vi "PID_linear.vi"(8 "Stop Controller Loop":bool) -> ()   [LabVIEW 2017]
uses:
  <vilib>/Platform/TimedLoop/XDataNode/timing_clust.ctl
  <vilib>/Platform/TimedLoop/XDataNode/nitl_modes.ctl
  <vilib>/Platform/TimedLoop/XDataNode/wakeup.ctl
  <vilib>/platform/TimedLoop/XDataNode/XDataNode.xnode
  <vilib>/Platform/TimedLoop/XDataNode/XDNodeRunTimeDep.lvlib
panel:
  in  "Starting Actuation State":dbl
  out "PID Actuations":dbl[](graph)
  in  "Actuation Min":dbl
  in  "Actuation Max":dbl
  out "Error":dbl
  out "Feedback":dbl
  out "Setpoint":dbl
  out "Saturated":bool
  out "Derivative State":dbl
  in  "Step Smoothing":dbl
  in  "Derivitative Max":dbl
  in  "D Gain":dbl
  out "Anti Windup":bool
  out "Integrator State":dbl
  in  "Integrator Min":dbl
  in  "Integrator Max":dbl
  in  "I Gain":dbl
  in  "P Gain":dbl
  # "PID Control"
  # "Proportional Control"
  # "Actuation Limits"
  # "Anti Windup Strategy"
  # "If the calcuated Actuation exceeds the Actuation Max or the Actuation Min, the Integrator State will only be allowed to accumulate in the direction of the allowed Actuation range and the Actuation will be saturated.\n\nIf the calculated Integrator State will be saturated to either the Integrator Max or Integrator Min."
  # "Integral Control"
  # "Integral Control"
  # "Derivative Smoothing Strategy"
  # "The derivative is calculated every n steps provide in the Step Smoothing Numeric Control for derivative smoothing."
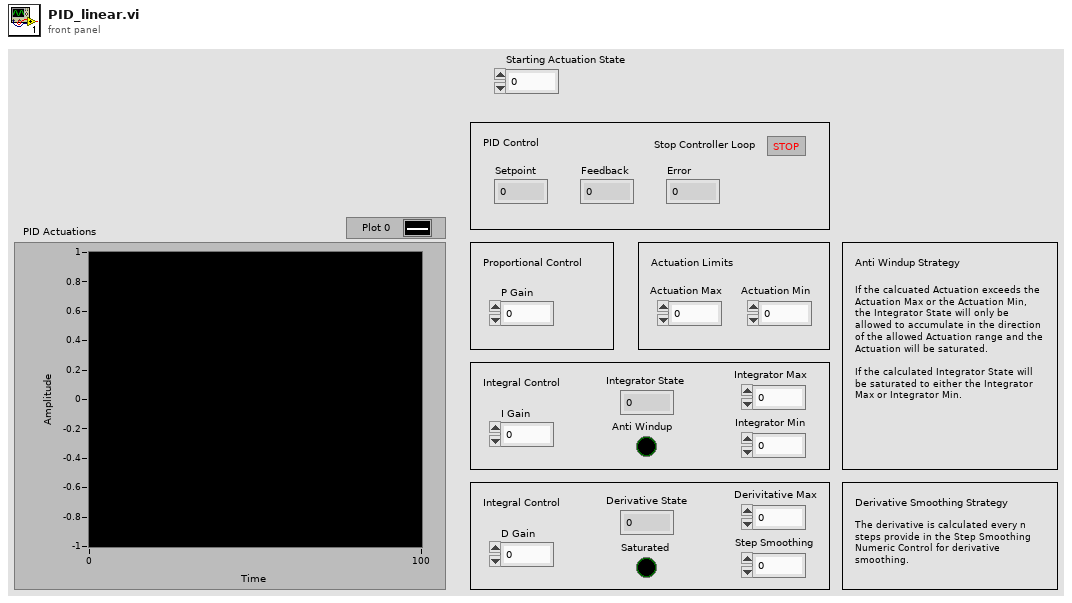
[diagram p1: front panel]
types:
  T1 = typedef "XDNodeRunTimeDep.lvlib/timing_clust.ctl" = cluster{"Expected End [f-1]":u64, "Actual End [f-1]":u64, "Finished Late? [f-1]":bool, "Expected End [i-1]":u64, "Actual End [i-1]":u64, "Finished Late? [i-1]":bool, "Expected Start [i]":u64, "Actual Start [i]":u64, "Expected Start [f]":u64, "Actual Start [f]":u64, "Source Name":string, "Structure Name":string, "Period":i64, "Deadline":i64, "Offset":i64, "Start":i64, "Priority":i32, "Timeout":i32, "Mode":T2, "Wakeup Reason":T3, "Error":errorcluster, "Source Type":string, "Secondary Source Type":string, "Global End Time":u64, "Global Start Time":u64, "Frame Duration":u64, "Iteration Duration":u64, "Assigned CPU":i32, "I/O Scan Engine Mode":u32}
  T2 = typedef "XDNodeRunTimeDep.lvlib/nitl_modes.ctl" = enum32{"No Change", "Process missed periods, maintain original phase", "Discard missed periods, maintain original phase", "Process missed periods, ignore original phase", "Discard missed periods, ignore original phase"}
  T3 = typedef "XDNodeRunTimeDep.lvlib/wakeup.ctl" = enum32{"Normal", "Aborted", "Asynchronous wakeup", "Timing source error", "Timed loop error", "Timeout"}
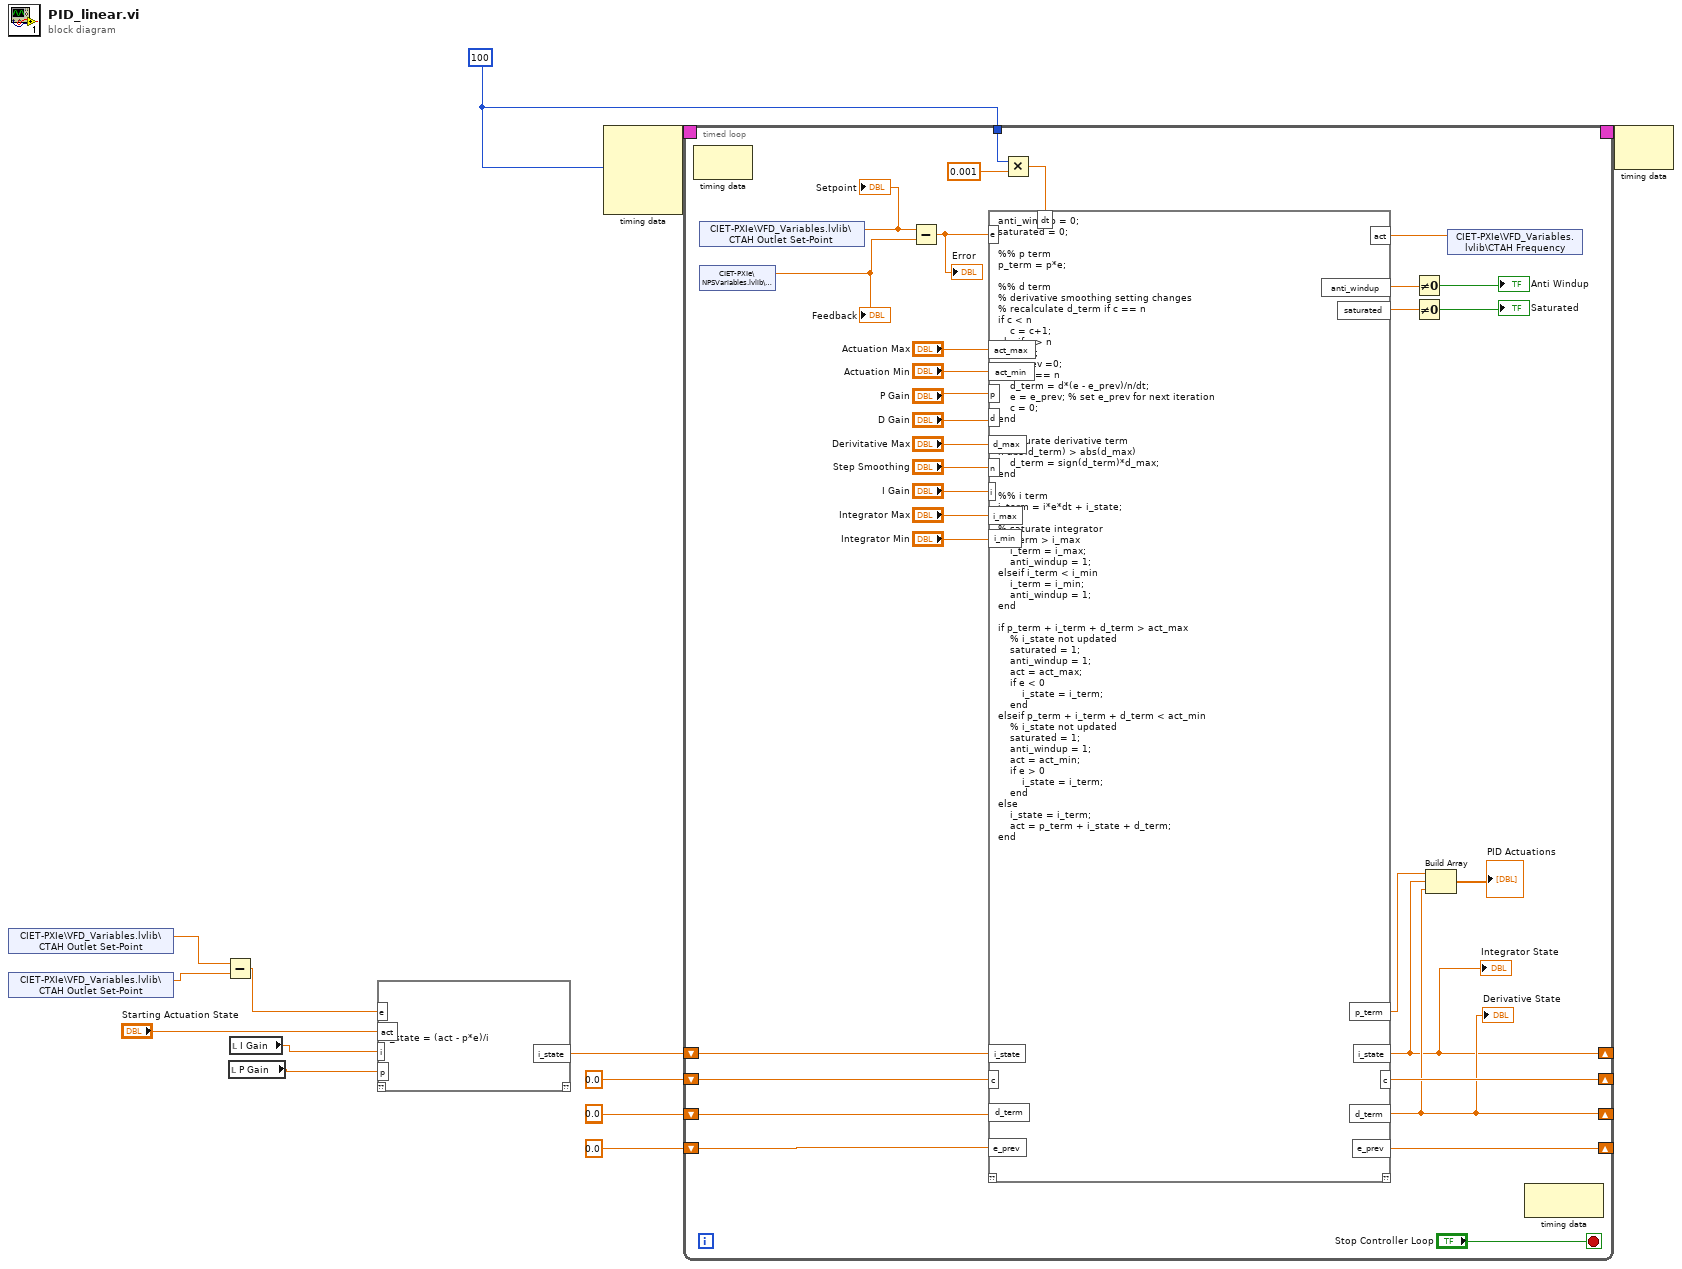
[diagram p0: block diagram]
diagram:
  w8 = 100
  (unwired) 0.0
  n1 = shared-variable "CIET-PXIe\\VFD_Variables.lvlib\\CTAH Outlet Set-Point"() -> (w4:dbl)  [unwired: 1 in, 1 out]
  n2 = shared-variable "CIET-PXIe\\VFD_Variables.lvlib\\CTAH Outlet Set-Point"() -> (w5:dbl)  [unwired: 1 in, 1 out]
  n3 = Subtract(x=w4, y=w5) -> (x-y=w3:dbl)
  n4 = local read "P Gain"() -> (w2:dbl)
  n5 = local read "I Gain"() -> (w1:dbl)
  n6 = script code="i_state = (act - p*e)/i"("e"=w3, "i"=w1, "act"="Starting Actuation State", "p"=w2) -> ("i_state"=w6:dbl)  [unwired: 1 in, 1 out]
  n7 = node-c288(w8) -> (w13:T1)  [unwired: 3 in]
  n8 = timed-loop {
    timing: w13 -> [_]
    timing-out: [_] -> w12
    shift-right: [w24] -> _
    shift-left: w6 -> [w33]
    shift-right: [w28] -> _
    shift-left: 0.0 -> [w32]
    shift-right: [w25] -> _
    shift-left: 0.0 -> [w31]
    shift-right: [w29] -> _
    shift-left: 0.0 -> [w30]
    tunnel: w8 -> [w20]
    stop <- "Stop Controller Loop" stop-if-true
    n9 = node-c288() -> ()  [unwired: 1 in, 1 out]
    n10 = shared-variable "CIET-PXIe\\VFD_Variables.lvlib\\CTAH Outlet Set-Point"() -> (w15:dbl)  [unwired: 1 in, 1 out]
    "Setpoint" <- w15
    n11 = shared-variable "CIET-PXIe\\NPSVariables.lvlib\\BT-41"() -> (w14:sgl)  [unwired: 1 in, 1 out]
    "Feedback" <- w14
    n12 = Subtract(x=w15, y=w14) -> (x-y=w27:dbl)
    "Error" <- w27
    n13 = Multiply(x=w20, y=0.001) -> (x*y=w21:dbl)
    n14 = script code="anti_windup = 0;\nsaturated = 0;\n\n%% p term\np_term = p*e;\n\n%% d term\n% derivative smoothing setting changes\n% recalculate d_term if c == n\nif c < n\n    c = c+1;\nelseif c > n \n    c = 0;\n    e_prev =0;\nelseif c == n\n    d_term = d*(e - e_prev)/n/dt;\n    e = e_prev; % set e_prev for next iteration\n    c = 0;\nend\n\n% saturate derivative term\nif abs(d_term) > abs(d_max)\n    d_term = sign(d_term)*d_max;\nend\n\n%% i term\ni_term = i*e*dt + i_state;\n\n% saturate integrator\nif i_term > i_max\n    i_term = i_max;\n    anti_windup = 1;\nelseif i_term < i_min\n    i_term = i_min;\n    anti_windup = 1;\nend\n\nif p_term + i_term + d_term > act_max\n    % i_state not updated\n    saturated = 1;\n    anti_windup = 1;\n    act = act_max;\n    if e < 0\n        i_state = i_term;\n    end\nelseif p_term + i_term + d_term < act_min\n    % i_state not updated\n    saturated = 1;\n    anti_windup = 1;\n    act = act_min;\n    if e > 0\n        i_state = i_term;\n    end\nelse\n    i_state = i_term;\n    act = p_term + i_state + d_term;\nend"("act_max"="Actuation Max", "act_min"="Actuation Min", "p"="P Gain", "d"="D Gain", "d_max"="Derivitative Max", "n"="Step Smoothing", "i"="I Gain", "i_max"="Integrator Max", "i_min"="Integrator Min", "i_state"=w33, "e_prev"=w30, "dt"=w21, "e"=w27, "c"=w32, "d_term"=w31) -> ("i_state"=w24:dbl, "e_prev"=w29:dbl, "anti_windup"=w43:dbl, "saturated"=w44:dbl, "act"=w18:dbl, "d_term"=w25:dbl, "c"=w28:dbl, "p_term"=w23:dbl)  [unwired: 1 in, 1 out]
    "Integrator State" <- w24
    "Derivative State" <- w25
    n15 = Not Equal To 0?(x=w43) -> (x != 0?=→"Anti Windup":bool)
    n16 = Not Equal To 0?(x=w44) -> (x != 0?=→"Saturated":bool)
    n17 = Build Array(w23, w24, w25) -> (→"PID Actuations":dbl[])
    n18 = shared-variable "CIET-PXIe\\VFD_Variables.lvlib\\CTAH Frequency"(w18) -> ()  [unwired: 1 in, 1 out]
    n19 = node-c288() -> ()  [unwired: 1 in, 1 out]
  }
  n20 = node-c288(w12) -> ()  [unwired: 1 out]
